vi "Parse Contained Variables.vi"(11 "String":string="${case${select}.addr}+${protocol}://${ip}:${port}") -> (3 "Contained Variables":string[](array[string]))   [LabVIEW 2017, in "INI-Static-Variable-Support.lvlib"]
uses:
  INI-Static-Variable-Support.lvlib
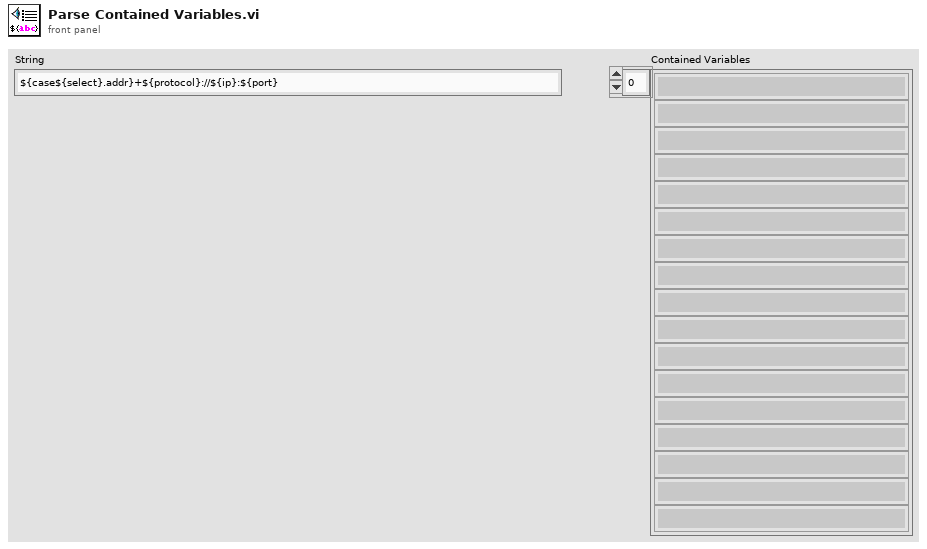
[diagram p1: front panel]
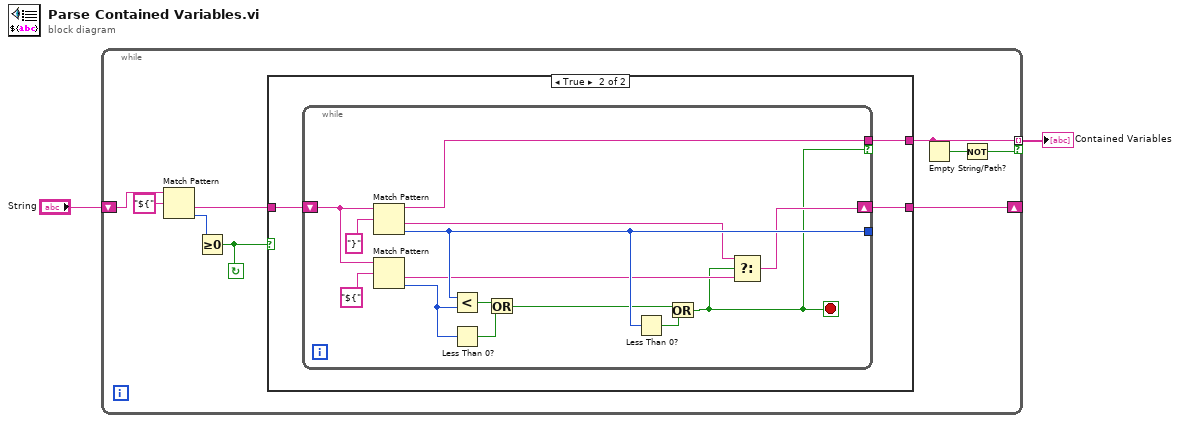
[diagram p0: block diagram]
diagram:
  n1 = while {
    shift-right: [w10] -> _
    shift-left: "String" -> [w11]
    tunnel: [w7] -> w1 mode=indexing if=w6
    stop <- w9 continue-if-true
    n2 = Match Pattern(string=w11, regular expression="${") -> (after substring=w3:string, offset past match=w4:i32)  [unwired: 1 in, 2 out]
    n3 = Greater Or Equal To 0?(x=w4) -> (x >= 0?=w9:bool)
    n4 = case shown="True" w9 {
      tunnel: w3 -> [w12 w15]
      tunnel: [w12 w14] -> w10
      tunnel: [_ w13] -> w7
      frame False {
      }
      frame True {
        n5 = while {
          tunnel: [w23] -> _
          shift-right: [w18] -> w14
          shift-left: w15 -> [w27]
          tunnel: [w17] -> w13 if=w16
          stop <- w16 stop-if-true
          n6 = Match Pattern(string=w27, regular expression="}") -> (before substring=w17:string, after substring=w19:string, offset past match=w23:i32)  [unwired: 1 in, 1 out]
          n7 = Match Pattern(string=w27, regular expression="${") -> (after substring=w20:string, offset past match=w24:i32)  [unwired: 1 in, 2 out]
          n8 = Less?(x=w23, y=w24) -> (x < y?=w26:bool)
          n9 = Less Than 0?(x=w24) -> (x < 0?=w21:bool)
          n10 = Or(x=w26, y=w21) -> (x .or. y?=w22:bool)
          n11 = Less Than 0?(x=w23) -> (x < 0?=w25:bool)
          n12 = Or(x=w22, y=w25) -> (x .or. y?=w16:bool)
          n13 = Select(t=w19, s=w16, f=w20) -> (s? t:f=w18:string)
        }
      }
    }
    n14 = Empty String/Path?(string/path=w7) -> (empty?=w8:bool)
    n15 = Not(x=w8) -> (.not. x?=w6:bool)
  }
  "Contained Variables" <- w1
